vi "Blob ReadData.vi"   [LabVIEW 2020, in "OpenLvVision_OpenCv.lvlib" / "Blob.lvclass"]
doc: "Retruns the data that is stored as nchw array inside the blob."
uses:
  Blob.lvclass
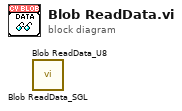
[diagram p0: block diagram]
diagram:
  n1 = call "Blob ReadData_SGL.vi"() -> ()  [unwired: 9 in, 3 out]
  n2 = call "Blob ReadData_U8.vi"() -> ()  [unwired: 9 in, 3 out]
